vi "pulse energy.vi"(8 "error in (no error)":errorcluster, 9 "Boolean":bool, 10 "handle":i32, 11 "Spectrum":cluster{dbl[], dbl[]}(graph)) -> (0 "error out":errorcluster, 1 "MaxPulse":cluster{i32[], dbl[]}(graph) caption="Spectrum", 2 "Pulse_time":dbl format="%.2f", 3 "PulseEnergy":dbl format="%#_12g", 5 "Pulse End":dbl format="%.4f", 7 "Pulse Begin":dbl format="%.4f")   [LabVIEW 2018]
uses:
  Program Files/National Instruments/LabVIEW 2018/user.lib/Gigahertz-Optik/GOMDTR9600/GOMDTR9600.lvlib
panel:
  out "Max index":i32
  out "Max value":dbl
  out "MAX_PULSE":dbl[](array[numeric])
  out "End index":i32
  out "End":dbl
  out "Begin index":i32
  out "Begin":dbl
  out "output array":dbl[][](array[numeric])
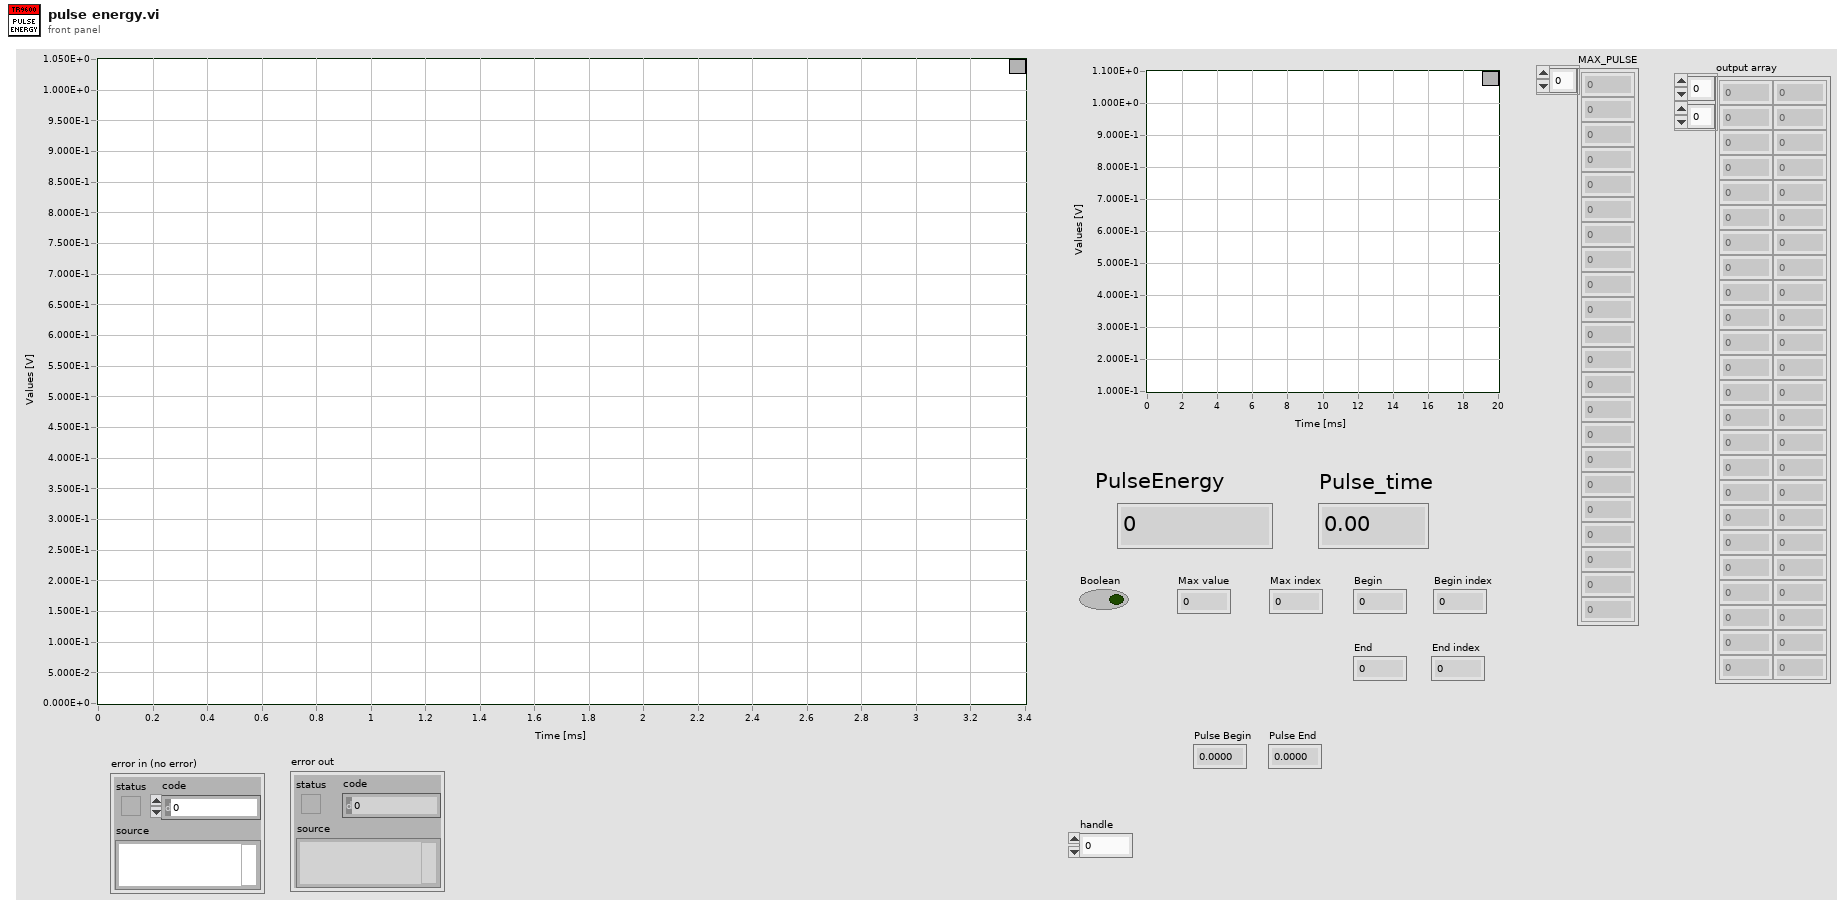
[diagram p1: front panel]
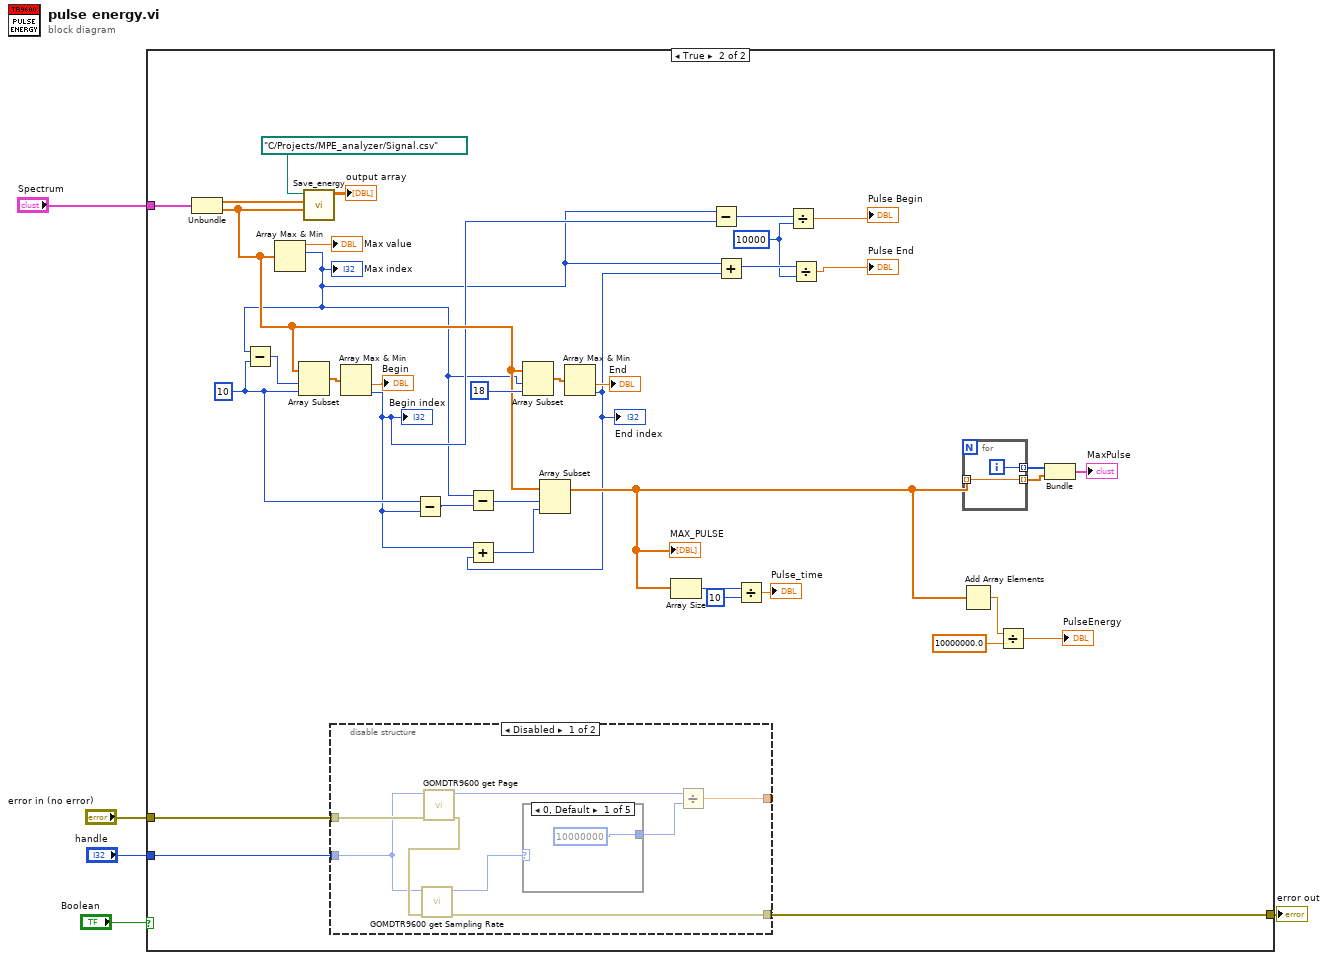
[diagram p0: block diagram]
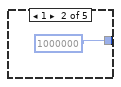
[diagram p3: hidden frame]
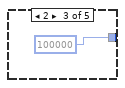
[diagram p4: hidden frame]
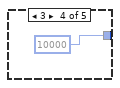
[diagram p5: hidden frame]
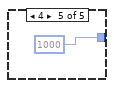
[diagram p6: hidden frame]
diagram:
  n1 = case shown="True" "Boolean" {
    tunnel: "handle" -> [_ w40]
    tunnel: "error in (no error)" -> [_ w42]
    tunnel: [_ w41] -> w3
    tunnel: "Spectrum" -> [_ w39]
    frame False {
    }
    frame True {
      w11 = 10000 ("y")
      w19 = 10 ("y")
      n2 = Unbundle(w39) -> (w25:dbl[], w23:dbl[])
      n3 = Array Max & Min(array=w23) -> (max value=→"Max value":dbl, max index (indices)=w15:i32)  [unwired: 2 out]
      "Max index" <- w15
      n4 = Subtract(x=w15, y=w19) -> (x-y=w33:i32)
      n5 = Array Subset(array=w23, index=w33, length=w19) -> (w38:dbl[])
      n6 = call "Save_energy.vi"("Voltage"=w23, "Time"=w25, "file path"=path "C:/Projects/MPE_analyzer/Signal.csv" ("file path (dialog if empty)")) -> ("output array"=→"output array":dbl[][])  [unwired: 8 in]
      n7 = disable-structure shown="Disabled" {
        disable-tunnel: w42 -> [w50 _]
        disable-tunnel: [w49 _] -> w41
        disable-tunnel: w40 -> [w44 _]
        disable-tunnel: [w43 _] -> _
        frame Disabled {
          n8 = call "GOMDTR9600 get Page.vi"("error in (no error)"=w50, "handle"=w44) -> ("error out"=w45:errorcluster, "value"=w47:i32)  [unwired: 7 in, 1 out]
          n9 = call "GOMDTR9600 get Sampling Rate.vi"("error in (no error)"=w45, "handle"=w44) -> ("error out"=w49:errorcluster, "value"=w48:i32)  [unwired: 7 in, 1 out]
          n10 = case shown="0, Default" w48 {
            tunnel: [10000000 ("value") 1000000 ("value") 100000 ("value") 10000 ("value") 1000 ("value")] -> w46
            frame 0, Default {
            }
            frame 1 {
            }
            frame 2 {
            }
            frame 3 {
            }
            frame 4 {
            }
          }
          n11 = Divide(x=w47, y=w46) -> (x/y=w43:dbl)
        }
        frame Enabled {
        }
      }
      n12 = Array Max & Min(array=w38) -> (min value=→"Begin":dbl, min index (indices)=w16:i32)  [unwired: 2 out]
      "Begin index" <- w16
      n13 = Subtract(x=w19, y=w16) -> (x-y=w18:i32)
      n14 = Subtract(x=w15, y=w18) -> (x-y=w32:i32)
      n15 = Array Subset(array=w23, index=w15, length=18 ("y")) -> (w36:dbl[])
      n16 = Array Max & Min(array=w36) -> (min value=→"End":dbl, min index (indices)=w14:i32)  [unwired: 2 out]
      "End index" <- w14
      n17 = Add(x=w16, y=w14) -> (x+y=w31:i32)
      n18 = Array Subset(array=w23, index=w32, length=w31) -> (w30:dbl[])
      "MAX_PULSE" <- w30
      n19 = Array Size(array=w30) -> (size(s)=w7:i32)
      n20 = Subtract(x=w15, y=w16) -> (x-y=w13:i32)
      n21 = Add(x=w15, y=w14) -> (x+y=w12:i32)
      n22 = Divide(x=w7, y=10) -> (x/y=→"Pulse_time":dbl)
      n23 = Divide(x=w13, y=w11) -> (x/y=→"Pulse Begin":dbl)
      n24 = Divide(x=w12, y=w11) -> (x/y=→"Pulse End":dbl)
      n25 = for {
        tunnel: w30 -> [w56] mode=indexing
        tunnel: [w57] -> w29 mode=indexing
        tunnel: [w56] -> w28 mode=indexing
        i -> [w57]
      }
      n26 = Add Array Elements(numeric array=w30) -> (sum=w21:dbl)
      n27 = Divide(x=w21, y=10000000.0) -> (x/y=→"PulseEnergy":dbl)
      n28 = Bundle(w29, w28) -> (→"MaxPulse":cluster{i32[], dbl[]})  [unwired: 1 in]
    }
  }
  "error out" <- w3
